vi "NML GPIB Data Log V0.5.vi"(0 "Point #":i32=-1) -> (1 "GPIB Data":dbl[](array[numeric]) format="%.2e", 2 "Stop":bool)   [LabVIEW 2025]
doc: "VI which calls the appropriate GPIB routines for a variety of instruments.\nScott Hannahs, NHMFL-FSU, Nov. 1993\nAuthor: Scott Hannahs <sth@magnet.fsu.edu>\n\nThis software is licensed for use under the “MIT License\"\nCopyright (c) 2025 Scott Hannahs, sth@sth@magnet.sthnet.net\n\nPermission is hereby granted, free of charge, to any person obtaining a copy of this software and associated documentation files (the \"Software\"), to deal in the Software without restriction, including without limitation the rights to use, copy, modify, merge, publish, distribute, sublicense, and/or sell copies of the Software, and to permit persons to whom the Software is furnished to do so, subject to the following conditions: The above copyright notice and this permission notice shall be included in all copies or substantial portions of the Software.\n\nTHE SOFTWARE IS PROVIDED \"AS IS\", WITHOUT WARRANTY OF ANY KIND, EXPRESS OR IMPLIED, INCLUDING BUT NOT LIMITED TO THE WARRANTIES OF MERCHANTABILITY, FITNESS FOR A PARTICULAR PURPOSE AND NONINFRINGEMENT. IN NO EVENT SHALL THE AUTHORS OR COPYRIGHT HOLDERS BE LIABLE FOR ANY CLAIM, DAMAGES OR OTHER LIABILITY, WHETHER IN AN ACTION OF CONTRACT, TORT OR OTHERWISE, ARISING FROM, OUT OF OR IN CONNECTION WITH THE SOFTWARE OR THE USE OR OTHER DEALINGS IN THE SOFTWARE."
uses:
  Sub Controls/NML GPIB List.ctl
panel:
  in  "LogCluster":T2={"McPherson Spectrometer Parameters"={"Instrument"=enum."AMI He Level Meter", "Grating Density"=4, "Parameters"=[500.0, 1.0, 600.0]}, "Wait at each Step"={"Instrument"=enum."Time Stamp", "GPIB Address"=1, "(Seconds)"=[1.0]}, "#1"={"Instrument"=enum."None", "GPIB Address"="", "Parameters"=[]}, "#2"={"Instrument"=enum."None", "GPIB Address"="", "Parameters"=[]}, "#3"={"Instrument"=enum."None", "GPIB Address"="", "Parameters"=[]}, "#4"={"Instrument"=enum."None", "GPIB Address"="", "Parameters"=[]}, "#5"={"Instrument"=enum."None", "GPIB Address"="", "Parameters"=[]}, "#6"={"Instrument"=enum."None", "GPIB Address"="", "Parameters"=[]}, "#7"={"Instrument"=enum."None", "GPIB Address"="", "Parameters"=[]}, "#8"={"Instrument"=enum."None", "GPIB Address"="", "Parameters"=[]}} {"#8"."Parameters" format="%.3e"; "#7"."Parameters" format="%.3e"; "#6"."Parameters" format="%.3e"; "#5"."Parameters" format="%.3e"; "#4"."Parameters" format="%.3e"; "#3"."Parameters" format="%.3e"; "#2"."Parameters" format="%.3e"; "#1"."Parameters" format="%.3e"; "McPherson Spectrometer Parameters"."Parameters" format="%.2f"; "McPherson Spectrometer Parameters"."Grating Density" items=["150", "300", "600", "1200", "1800"]; "Wait at each Step"."(Seconds)" format="%.1f"; "Wait at each Step"."GPIB Address" min=1 max=31 step=1}
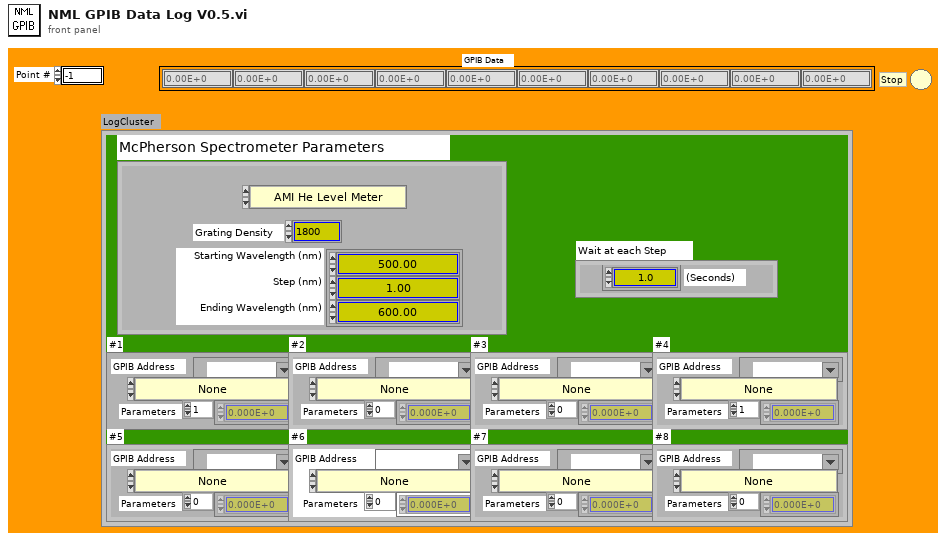
[diagram p1: front panel]
types:
  T1 = typedef "NML GPIB List.ctl" = enum16{"None", "Field", "Field - SCM1", "DMM", "DMM - HP 34401", "Keithley 2XXX", "Running DMM Ave", "Running HP34401", "Running K2XXX Ave", "SRS 830 - CH 1", "SRS 830 - CH1 & 2", "SRS PTC10", "Signal Rec 7265 - X", "Signal Rec 7265 - X&Y", "DRC 93C - Sample", "DRC 93C - Control", "DRC 93C - Sam&Con", "CryoCon Sensor A", "CryoCon Sensor B", "Cond 20C Sensor 1", "Cond 20C Sensor 2", "LS 336 Read", "LS 340 Read", "LS 370 Read", "LS 370 Select", "AVS 46 Bridge", "BLM Rotator Read Position", "Linear Research 700", "LR 700 Select", "Keithley 3330 - LCZ", "A-H Capacitance", "Digital Integrator", "SRS 400 Phot Ctr", "LakeShore VSM", "AMI He Level Meter", "Time Stamp", "Wait", "Invert Current", "K230 Linear V", "K230 VÅB^2", "Temp Ramp", "Power Ramp", "Freq Sweep", "LTC Stable T", "Scanner Step", "IMS Stepper Increment", "BLM Stepper Increment", "Omega CNi32"}
  T2 = cluster{"McPherson Spectrometer Parameters":cluster{"Instrument":T1, "Grating Density":u32, "Parameters":dbl[]}, "Wait at each Step":cluster{"Instrument":T1, "GPIB Address":u32, "(Seconds)":dbl[]}, "#1":cluster{"Instrument":T1, "GPIB Address":refnum<visa-resource-name>, "Parameters":dbl[]}, "#2":cluster{"Instrument":T1, "GPIB Address":refnum<visa-resource-name>, "Parameters":dbl[]}, "#3":cluster{"Instrument":T1, "GPIB Address":refnum<visa-resource-name>, "Parameters":dbl[]}, "#4":cluster{"Instrument":T1, "GPIB Address":refnum<visa-resource-name>, "Parameters":dbl[]}, "#5":cluster{"Instrument":T1, "GPIB Address":refnum<visa-resource-name>, "Parameters":dbl[]}, "#6":cluster{"Instrument":T1, "GPIB Address":refnum<visa-resource-name>, "Parameters":dbl[]}, "#7":cluster{"Instrument":T1, "GPIB Address":refnum<visa-resource-name>, "Parameters":dbl[]}, "#8":cluster{"Instrument":T1, "GPIB Address":refnum<visa-resource-name>, "Parameters":dbl[]}}
  T3 = cluster{"Instrument":T1, "GPIB Address":refnum<visa-resource-name>, "Parameters":dbl[]}
  T4 = cluster{"#1":cluster{"Instrument":T1, "GPIB Address":refnum<visa-resource-name>, "Parameters":dbl[]}, "#2":cluster{"Instrument":T1, "GPIB Address":refnum<visa-resource-name>, "Parameters":dbl[]}, "#3":cluster{"Instrument":T1, "GPIB Address":refnum<visa-resource-name>, "Parameters":dbl[]}, "#4":cluster{"Instrument":T1, "GPIB Address":refnum<visa-resource-name>, "Parameters":dbl[]}, "#5":cluster{"Instrument":T1, "GPIB Address":refnum<visa-resource-name>, "Parameters":dbl[]}, "#6":cluster{"Instrument":T1, "GPIB Address":refnum<visa-resource-name>, "Parameters":dbl[]}, "#7":cluster{"Instrument":T1, "GPIB Address":refnum<visa-resource-name>, "Parameters":dbl[]}, "#8":cluster{"Instrument":T1, "GPIB Address":refnum<visa-resource-name>, "Parameters":dbl[]}}
  T5 = cluster{"Instrument":T1, "GPIB Address":refnum<visa-resource-name>, "Parameters":dbl[]}[]
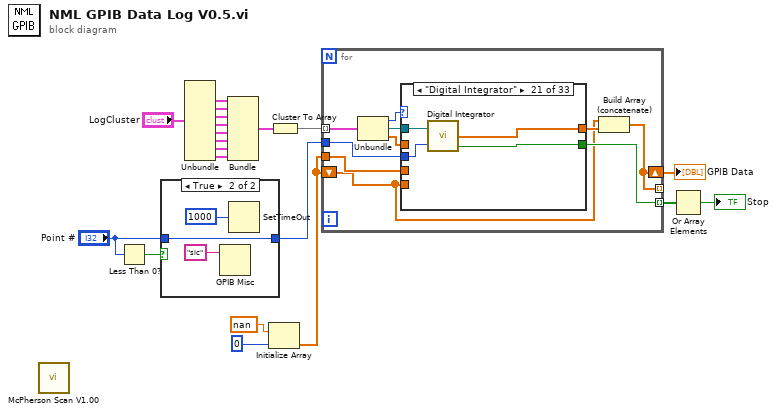
[diagram p0: block diagram]
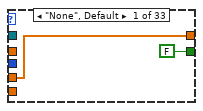
[diagram p2: hidden frame]
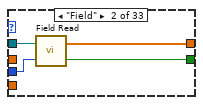
[diagram p3: hidden frame]
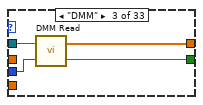
[diagram p4: hidden frame]
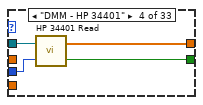
[diagram p5: hidden frame]
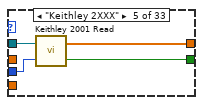
[diagram p6: hidden frame]
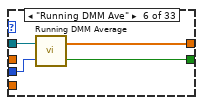
[diagram p7: hidden frame]
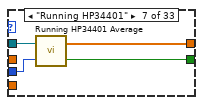
[diagram p8: hidden frame]
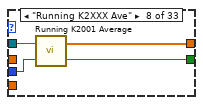
[diagram p9: hidden frame]
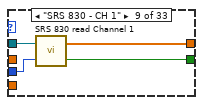
[diagram p10: hidden frame]
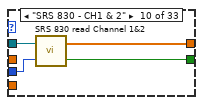
[diagram p11: hidden frame]
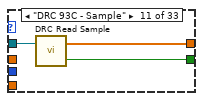
[diagram p12: hidden frame]
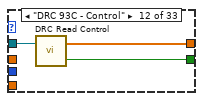
[diagram p13: hidden frame]
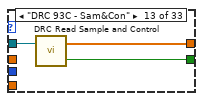
[diagram p14: hidden frame]
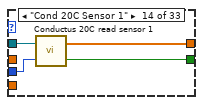
[diagram p15: hidden frame]
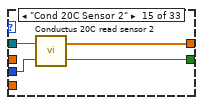
[diagram p16: hidden frame]
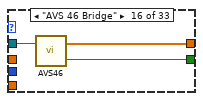
[diagram p17: hidden frame]
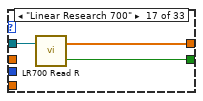
[diagram p18: hidden frame]
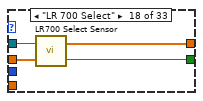
[diagram p19: hidden frame]
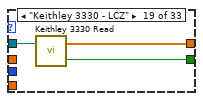
[diagram p20: hidden frame]
diagram:
  n1 = call "McPherson Scan V1.00.vi"() -> ()  [unwired: 5 in, 2 out]
  n2 = Less Than 0?(x="Point #") -> (x < 0?=w16:bool)
  n3 = case shown="True" w16 {
    tunnel: [w21 w23] -> w12
    tunnel: "Point #" -> [w21 w23]
    frame False {
    }
    frame True {
      n4 = GPIB Misc(0:"sic" ("command string")) -> ()  [unwired: 1 in, 3 out]
      n5 = SetTimeOut(1:1000 ("new timeout (10000)")) -> ()  [unwired: 1 out]
    }
  }
  n6 = Unbundle("LogCluster") -> ("#1"=w8:T3, "#2"=w7:T3, "#3"=w6:T3, "#4"=w5:T3, "#5"=w4:T3, "#6"=w3:T3, "#7"=w2:T3, "#8"=w1:T3)  [unwired: 2 out]
  n7 = Bundle("#1"=w8, "#2"=w7, "#3"=w6, "#4"=w5, "#5"=w4, "#6"=w3, "#7"=w2, "#8"=w1) -> (w9:T4)  [unwired: 1 in]
  n8 = Initialize Array(nan, 0) -> (w14:dbl[])
  n9 = Cluster To Array(cluster=w9) -> (array=w13:T5)
  n10 = for {
    shift-right: [w34] -> w10
    shift-left: w14 -> [w25]
    tunnel: w12 -> [w29]
    tunnel: w13 -> [w30] mode=indexing
    tunnel: [w28] -> w11 mode=indexing
    tunnel: w14 -> [w27]
    tunnel: [w34] -> _ mode=indexing
    n11 = Unbundle(w30) -> ("Instrument"=w31:T1, "GPIB Address"=w32:refnum<visa-resource-name>, "Parameters"=w26:dbl[])
    n12 = case shown="\"Digital Integrator\"" w31 {
      tunnel: [FALSE w39 w43 w47 w51 w55 w59 w63 w68 w72 w75 w78 w81 w84 w88 w91 w94 w98 w101 w105 w107 w113 w116 w118 w122 w127 w132 w137 w142 w147 w149 w155 w161] -> w28
      tunnel: w29 -> [_ w37 w41 w45 w49 w53 w57 w61 w65 w69 _ _ _ w82 w86 _ _ _ _ w103 w110 _ _ w120 w124 w125 w129 w135 w140 w145 w151 w156 w160]
      tunnel: [w35 w40 w44 w48 w52 w56 w60 w64 w67 w71 w74 w77 w80 w85 w89 w90 w93 w97 w100 w104 w108 w114 w117 w119 w123 w128 w133 w138 w143 w148 w150 w154 w162] -> w33
      tunnel: w32 -> [_ w38 w42 w46 w50 w54 w58 w62 w66 w70 w73 w76 w79 w83 w87 w92 w95 w99 w102 w106 w109 w112 w115 _ _ w126 w131 w136 w141 w146 w152 w157 w159]
      tunnel: w27 -> [w35 _ _ _ _ _ _ _ _ _ _ _ _ _ _ _ _ _ _ _ _ _ _ _ _ _ _ _ _ _ _ _ _]
      tunnel: w26 -> [_ _ _ _ _ _ _ _ _ _ _ _ _ _ _ _ _ w96 _ _ _ w111 _ _ w121 _ w130 _ w139 w144 _ w153 w158]
      tunnel: w25 -> [_ _ _ _ _ _ _ _ _ _ _ _ _ _ _ _ _ _ _ _ _ _ _ _ _ _ _ w134 _ _ _ _ _]
      frame "None", Default {
      }
      frame "Field" {
        n13 = call "Field Read.vi"("Point #"=w37, "Instrument Address"=w38) -> ("Stop"=w39:bool, "Field"=w40:dbl[])
      }
      frame "DMM" {
        n14 = call "DMM Read.vi"("Point #"=w41, "Instrument Address"=w42) -> ("Stop"=w43:bool, "Measurement"=w44:dbl[])
      }
      frame "DMM - HP 34401" {
        n15 = call "HP 34401 Read.vi"("Point #"=w45, "Instrument Address"=w46) -> ("Stop"=w47:bool, "Measurement"=w48:dbl[])
      }
      frame "Keithley 2XXX" {
        n16 = call "Keithley 2001 Read.vi"("Point #"=w49, "Instrument Address"=w50) -> ("Stop"=w51:bool, "Measurement"=w52:dbl[])
      }
      frame "Running DMM Ave" {
        n17 = call "Running DMM Average.vi"("Point #"=w53, "Instrument Address"=w54) -> ("Stop"=w55:bool, 1:w56:dbl[])
      }
      frame "Running HP34401" {
        n18 = call "Running HP34401 Average.vi"("Point #"=w57, "Instrument Address"=w58) -> ("Stop"=w59:bool, 1:w60:dbl[])
      }
      frame "Running K2XXX Ave" {
        n19 = call "Running K2001 Average.vi"("Point #"=w61, "Instrument Address"=w62) -> ("Stop"=w63:bool, 1:w64:dbl[])
      }
      frame "SRS 830 - CH 1" {
        n20 = call "SRS 830 read Channel 1.vi"("Point #"=w65, "Instrument Address"=w66) -> ("Stop"=w68:bool, "SRS 830 Output"=w67:dbl[])
      }
      frame "SRS 830 - CH1 & 2" {
        n21 = call "SRS 830 read Channel 1&2.vi"("Point #"=w69, "Instrument Address"=w70) -> ("Stop"=w72:bool, "SRS 830 Output"=w71:dbl[])
      }
      frame "DRC 93C - Sample" {
        n22 = call "DRC Read Sample.vi"("Instrument Address"=w73) -> ("Stop"=w75:bool, "Output"=w74:dbl[])  [unwired: 1 in]
      }
      frame "DRC 93C - Control" {
        n23 = call "DRC Read Control.vi"("Instrument Address"=w76) -> ("Stop"=w78:bool, "Output"=w77:dbl[])  [unwired: 1 in]
      }
      frame "DRC 93C - Sam&Con" {
        n24 = call "DRC Read Sample and Control.vi"("Instrument Address"=w79) -> ("Stop"=w81:bool, "Output"=w80:dbl[])  [unwired: 1 in]
      }
      frame "Cond 20C Sensor 1" {
        n25 = call "Conductus 20C read sensor 1.vi"("Point #"=w82, "Instrument Address"=w83) -> ("Stop"=w84:bool, "Output"=w85:dbl[])
      }
      frame "Cond 20C Sensor 2" {
        n26 = call "Conductus 20C read sensor 2.vi"("Point #"=w86, "Instrument Address"=w87) -> ("Stop"=w88:bool, "Output"=w89:dbl[])
      }
      frame "AVS 46 Bridge" {
        n27 = call "AVS46.vi"("Instrument Address"=w92) -> ("Stop"=w91:bool, "Measurement"=w90:dbl[])  [unwired: 1 in]
      }
      frame "Linear Research 700" {
        n28 = call "LR700 Read R.vi"("Instrument Address"=w95) -> ("Stop"=w94:bool, "Measurement"=w93:dbl[])  [unwired: 1 in]
      }
      frame "LR 700 Select" {
        n29 = call "LR700 Select Sensor.vi"("Parameters"=w96, "Instrument Address"=w99) -> ("Stop"=w98:bool, "Array"=w97:dbl[])
      }
      frame "Keithley 3330 - LCZ" {
        n30 = call "Keithley 3330 Read.vi"("Instrument Address"=w102) -> ("Stop"=w101:bool, "Measurement"=w100:dbl[])  [unwired: 1 in]
      }
      frame "A-H Capacitance" {
        n31 = call "A-H Cap.vi"("Point #"=w103, "Instrument Address"=w106) -> ("Stop"=w105:bool, "Measurement"=w104:dbl[])
      }
      frame "Digital Integrator" {
        n32 = call "Digital Integrator.vi"("Instrument Address"=w109, "Index"=w110) -> (3:w108:dbl[], "Stop"=w107:bool)  [unwired: 1 out]
      }
      frame "SRS 400 Phot Ctr" {
        n33 = call "SRS 400 Read.vi"("Parameters"=w111, "Instrument Address"=w112) -> ("Stop"=w113:bool, "Data"=w114:dbl[])
      }
      frame "LakeShore VSM" {
        n34 = call "LakeShore VSM 7300 EMU read.vi"("Instrument Address"=w115) -> ("Stop"=w116:bool, "Output"=w117:dbl[])  [unwired: 1 in]
      }
      frame "Time Stamp" {
        n35 = call "Time Stamp-old.vi"("Point #"=w120) -> ("Stop"=w118:bool, "Time Stamp (Sec)"=w119:dbl[])  [unwired: 1 in]
      }
      frame "Wait" {
        n36 = call "Seconds Wait.vi"("Point #"=w124, "Parameters"=w121) -> ("Stop"=w122:bool, "Time Stamp (Sec)"=w123:dbl[])
      }
      frame "Invert Current" {
        n37 = call "Invert Current Keithley 220.vi"("Point #"=w125, "Instrument Address"=w126) -> ("Stop"=w127:bool, "Keithley 220 Current"=w128:dbl[])  [unwired: 2 in]
      }
      frame "K230 Linear V" {
        n38 = call "Keithley 230 Voltage Ramp.vi"("Point #"=w129, "Parameters"=w130, "Instrument Address"=w131) -> ("Stop"=w132:bool, "Keithley 230 Voltage"=w133:dbl[])  [unwired: 1 in]
      }
      frame "K230 VÅB^2" {
        n39 = call "Keithley 230 V prop B^2.vi"("Point #"=w135, "GPIB Data In"=w134, "Instrument Address"=w136) -> ("Stop"=w137:bool, "Keithley 230 Voltage"=w138:dbl[])  [unwired: 1 in]
      }
      frame "Temp Ramp" {
        n40 = call "Conductus Ramp Temperature.vi"("Point #"=w140, "Parameters"=w139, "Instrument Address"=w141) -> ("Stop"=w142:bool, "Data Out"=w143:dbl[])  [unwired: 1 in]
      }
      frame "Power Ramp" {
        n41 = call "Conductus Ramp Power.vi"("Point #"=w145, "Parameters"=w144, "Instrument Address"=w146) -> ("Stop"=w147:bool, "Data Out"=w148:dbl[])  [unwired: 1 in]
      }
      frame "LTC Stable T" {
        n42 = call "LTC change to stable temp.vi"("Point Number"=w151, "L:TC 21 Address"=w152) -> ("Stop"=w149:bool, "Stable temperature (K)"=w150:dbl[])
      }
      frame "Scanner Step" {
        n43 = call "Scanme.vi"("Index"=w156, "Parameters"=w153, "Instrument Address"=w157) -> ("Stop"=w155:bool, "Array"=w154:dbl[])  [unwired: 1 in]
      }
      frame "AMI He Level Meter" {
        n44 = call "Parker Stepper Control.vi"("Point #"=w160, "Parameters"=w158, "Instrument Address"=w159) -> ("Stop"=w161:bool, "Data Out"=w162:dbl[])  [unwired: 1 in]
      }
    }
    n45 = Build Array (concatenate)(w25, w33) -> (w34:dbl[])
  }
  "GPIB Data" <- w10
  n46 = Or Array Elements(Boolean array=w11) -> (logical OR=→"Stop":bool)
